vi "display FC status.vi"(8 "error in":errorcluster={"status"=FALSE, "code"=-1950679034, "source"="Shared Variable in Large VAC READBACKS.vi<APPEND>\nThis error or warning occurred while reading the following Shared Variable:\n\\\\My Computer\\lowendshmc\\digital outputs\n\\\\192.168.1.200\\lowendshmc\\digital outputs"}, 9 "FC Status":T1, 10 "Actuator":bool=TRUE, 11 "FC display Refnum":refnum<vi>) -> (0 "error out":errorcluster={"status"=FALSE, "code"=-1950679034, "source"="Shared Variable in Large VAC READBACKS.vi<APPEND>\nThis error or warning occurred while reading the following Shared Variable:\n\\\\My Computer\\lowendshmc\\digital outputs\n\\\\192.168.1.200\\lowendshmc\\digital outputs"})   [LabVIEW 2016]
doc: "controls the display of if a cup or apt. is in the beamline"
uses:
  Controls/Faraday cup states.ctl
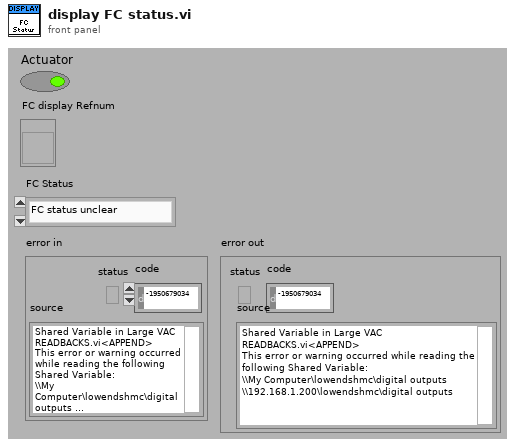
[diagram p1: front panel]
types:
  T1 = typedef "Faraday cup states.ctl" = enum16{"FC status unclear", "FC in", "FC out"}
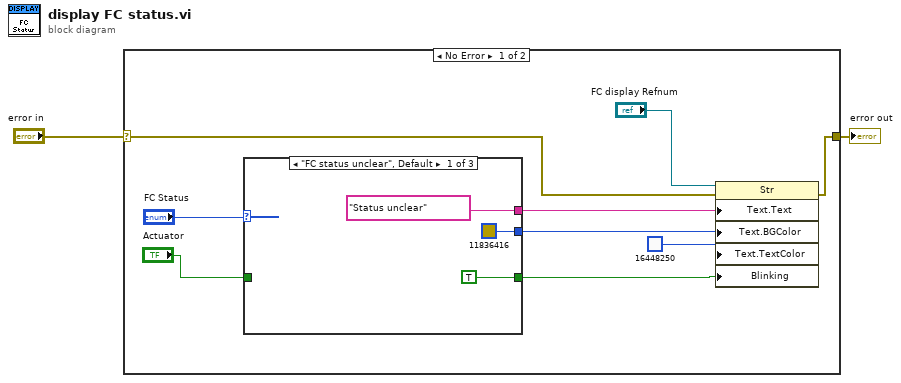
[diagram p0: block diagram]
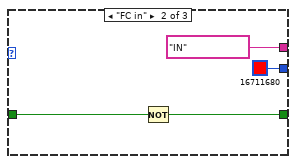
[diagram p2: hidden frame]
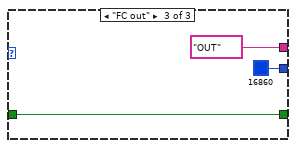
[diagram p3: hidden frame]
diagram:
  n1 = case shown="No Error" "error in" {
    selector: "error in" -> [w5 w22]
    tunnel: [w7 w22] -> w2
    frame No Error {
      n2 = case shown="\"FC status unclear\", Default" "FC Status" {
        tunnel: ["Status unclear" ("Text.Text") "IN" ("Text.Text") "OUT" ("Text.Text")] -> w9
        tunnel: [u32 11836416 u32 16711680 u32 16860] -> w10
        tunnel: [TRUE w15 w19] -> w4
        tunnel: "Actuator" -> [_ w16 w19]
        frame "FC status unclear", Default {
        }
        frame "FC in" {
          n3 = Not(x=w16) -> (.not. x?=w15:bool)
        }
        frame "FC out" {
        }
      }
      n4 = property on="Property Node" class="Str"(reference="FC display Refnum", error in=w5, "Text.Text"=w9, "Text.BGColor"=w10, "Text.TextColor"=u32 16448250, "Blinking"=w4) -> (error out=w7:errorcluster)  [unwired: 1 out]
    }
    frame Error {
    }
  }
  "error out" <- w2
